vi "Process.vi"(8 "error in":errorcluster, 11 "Measurement.Free":refnum<class "Measurement.Free.lvclass">) -> (0 "error out":errorcluster, 3 "Measurement.Free out":refnum<class "Measurement.Free.lvclass">)   [LabVIEW 2017, in "Measurement.Free.lvclass"]
doc: "---------------------------------------------------------------\nJKI State Machine Objects™\nhttp://jki.net/state-machine-objects/\nCopyright (C) 2005-2015, JKI <info@jki.net>\nALL RIGHTS RESERVEDJKI State Machine Objects (SMO) 1.0.0.5\nJKI - JKI\nCopyright (c) 2016, JKI"
uses:
  Measurement.Free.lvclass
  D:/Program Files (x86)/National Instruments/LabVIEW 2017/vi.lib/JKI/JKI SMO/SMO/SMO.lvclass
  D:/upwork/Laser Measurement Tool/Laser/project/Subsystems/Measurement/Measurement.lvclass
  <vilib>/JKI/JKI SMO/SMO/Typedefs/SMOState --Enum.ctl
  <vilib>/JKI/JKI SMO/SMO/Typedefs/Parent Call--Enum.ctl
  Measurement/Typedefs/Measurement.State--Enum.ctl
  Typedefs/Measurement.Free.Device--Enum.ctl
  Typedefs/Measurement.Free.Measured--Data.ctl
  OPA/Typedefs/OPA.Parameter--Enum.ctl
  Measurement/Typedefs/PublicEvents--Measurement.Initialized.ctl
  Measurement/Typedefs/PublicEvents--Measurement.Escaped.ctl
  SMU/SMU.lvclass
  D:/upwork/Laser Measurement Tool/Laser/project/Subsystems/MeasuringDevice/MeasuringDevice.lvclass
  LIA/LIA.lvclass
  OPM/OPM.lvclass
  Measurement/Measurement.lvclass
  <vilib>/JKI/JKI SMO/SMO/SMO.lvclass
  MeasuringDevice/MeasuringDevice.lvclass
  OPA/OPA.lvclass
panel:
  out "LIA GUID":string
  out "SMU GUID":string
  out "LIA Name":string
  out "SMU Name":string
  out "LIA State":T1
  out "SMU State":T1
  # "Measurement.Free\nProcess.vi"
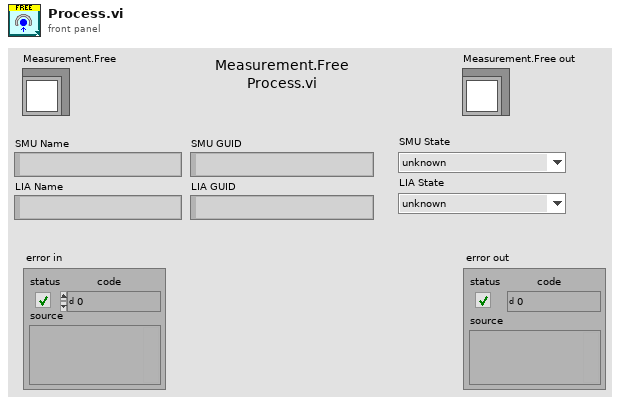
[diagram p1: front panel]
types:
  T1 = typedef "SMO.lvclass/SMOState --Enum.ctl" = enum16{"unknown", "Created", "Started", "Stopped"}
  T2 = typedef "SMO.lvclass/Parent Call--Enum.ctl" = enum16{"Allows parent to run", "Does not request parent to run"}
  T3 = typedef "Measurement.lvclass/Measurement.State--Enum.ctl" = enum16{"Uninitialized", "Initialized", "Started", "Paused", "Stopped"}
  T4 = typedef "Measurement.Free.lvclass/Measurement.Free.Device--Enum.ctl" = enum16{"SMU", "LIA", "OPM", "OPA"}
  T5 = enum32{"invalid app kind", "Development System", "Run Time System", "Student Edition", "Embedded LabVIEW", "Evaluation", "Custom"}
  T6 = enum32{"Invalid", "Standard", "Closed", "Hidden", "Minimized", "Maximized"}
  T7 = typedef "Measurement.lvclass/PublicEvents--Measurement.Initialized.ctl" = bool
  T8 = typedef "Measurement.lvclass/PublicEvents--Measurement.Escaped.ctl" = bool
  T9 = typedef "Measurement.Free.lvclass/Dependencies--Cluster.ctl" = cluster{"SMU":refnum<class "SMU.lvclass">, "LIA":refnum<class "LIA.lvclass">, "OPM":refnum<class "OPM.lvclass">, "OPA":refnum<class "OPA.lvclass">}
  T10 = typedef "Measurement.Free.lvclass/Configuration--Cluster.ctl" = cluster{"Measurement.Type":T11, "Hardware":T12}
  T11 = typedef "Measurement.lvclass/Measurement.Type--Enum.ctl" = enum16{"Free", "I/V Curve", "Wavelength sweeping", "Photocurrent mapping"}
  T12 = typedef "Measurement.Free.lvclass/Configuration.Hardware--Cluster.ctl" = cluster{"SMU":T13, "LIA":T15, "OPM":T17, "OPA":T19}
  T13 = typedef "Measurement.lvclass/Configuration.SMU--Cluster.ctl" = cluster{"Enable":bool, "SMU Model":string, "Configuration":T14}
  T14 = typedef "SMU.lvclass/Configuration--Cluster.ctl" = cluster{"VISA Resource":string, "Channel":string}
  T15 = typedef "Measurement.lvclass/Configuration.LIA--Cluster.ctl" = cluster{"Enable":bool, "LIA Model":string, "Configuration":T16}
  T16 = typedef "LIA.lvclass/Configuration--Cluster.ctl" = cluster{"VISA Resource":string}
  T17 = typedef "Measurement.lvclass/Configuration.OPM--Cluster.ctl" = cluster{"Enable":bool, "OPM Model":string, "Configuration":T18}
  T18 = typedef "OPM.lvclass/Configuration--Cluster.ctl" = cluster{"VISA Resource":string}
  T19 = typedef "Measurement.lvclass/Configuration.OPA--Cluster.ctl" = cluster{"Enable":bool, "OPA Model":string, "Configuration":T20}
  T20 = typedef "OPA.lvclass/Configuration--Cluster.ctl" = cluster{"Serial Number":string}
  T21 = cluster{"Core":cluster{"Current VI Reference":refnum<vi>, "Close Panel on Exit?":bool, "error":errorcluster}, "Self Reference":refnum<class "Measurement.Free.lvclass">, "Dependencies":T9, "Configuration":T10, "Initialized":bool, "State":T3, "SMU Completed":bool, "LIA Completed":bool, "OPM Completed":bool}
  T22 = typedef "Measurement.Free.lvclass/PrivateEvents--Measurement.Free.SMU.SetVoltage.ctl" = dbl
  T23 = typedef "Measurement.Free.lvclass/PrivateEvents--Measurement.Free.OPA.SetWavelength.ctl" = dbl
  T24 = typedef "Measurement.Free.lvclass/PrivateEvents--Measurement.Free.OPA.SetShutterState.ctl" = bool
  T25 = typedef "Measurement.Free.lvclass/Measurement.Free.Measured--Data.ctl" = cluster{"Device":T4, "Parameter":variant, "Data":variant}
  T26 = typedef "OPA.lvclass/OPA.Parameter--Enum.ctl" = enum16{"Wavelength", "Shutter State"}
  T27 = cluster{"Current VI Reference":refnum<vi>, "Close Panel on Exit?":bool, "error":errorcluster}
  T28 = typedef "SMO.lvclass/Protected Events.ctl" = cluster{"StopProcesses":refnum<user-event>, "AbortProcesses":refnum<user-event>, "Config Changed":refnum<user-event>, "Dependency":refnum<user-event>}
  T29 = typedef "Measurement.Free.lvclass/PrivateEvents--Cluster.ctl" = cluster{"SMU.SetVoltage":refnum<user-event>, "OPA.SetWavelength":refnum<user-event>, "OPA.SetShutterState":refnum<user-event>}
  T30 = typedef "SMO.lvclass/Public Events.ctl" = cluster{"Error":refnum<user-event>, "State":refnum<user-event>, "Reserve State":refnum<user-event>}
  T31 = cluster{"Event Registration Refnum":refnum<event-registration>, "Measurement Protected Events":refnum<event-registration>, "SMU Public Events":refnum<event-registration>, "LIA Public Events":refnum<event-registration>, "OPM Public Events":refnum<event-registration>, "OPA Public Events":refnum<event-registration>}
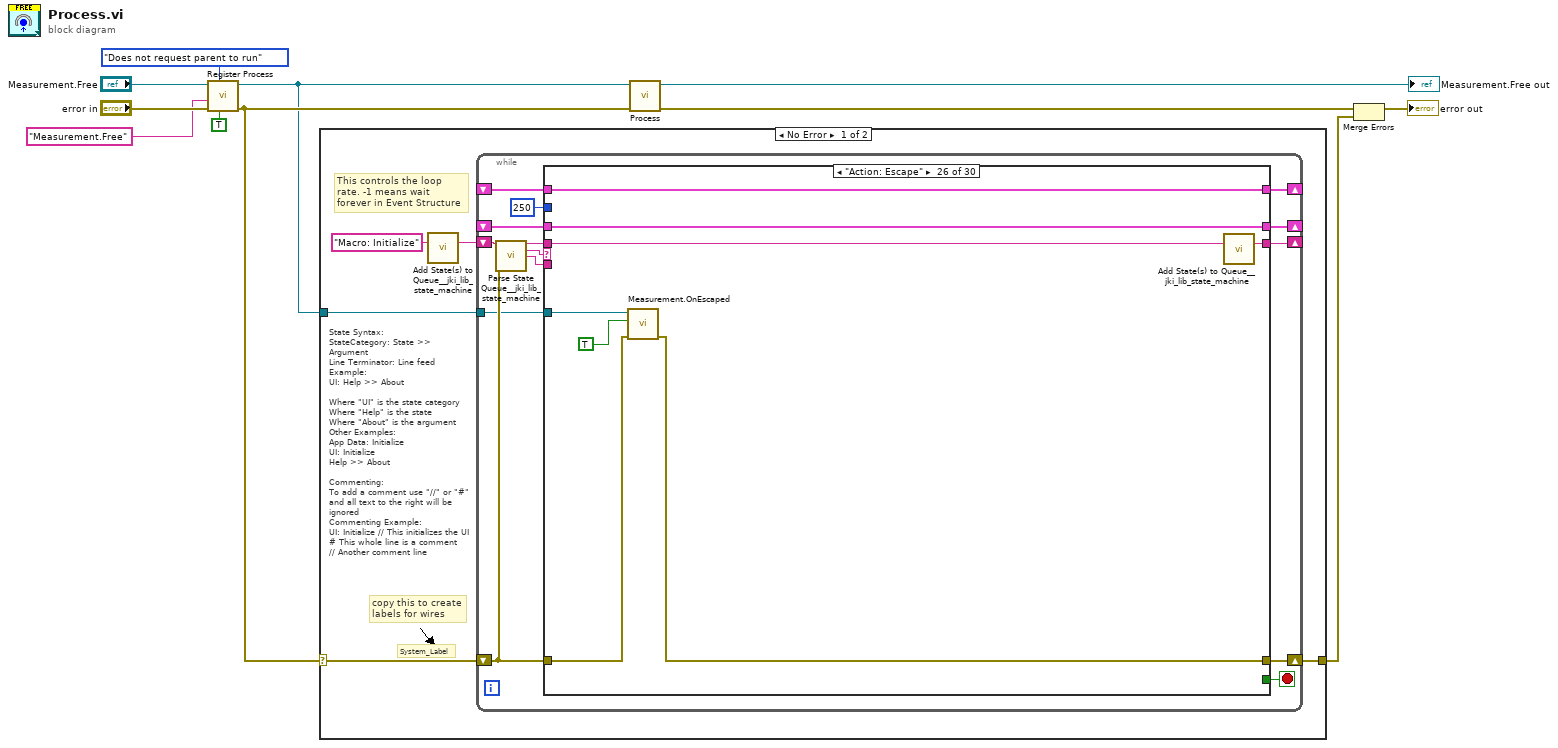
[diagram p0: block diagram]
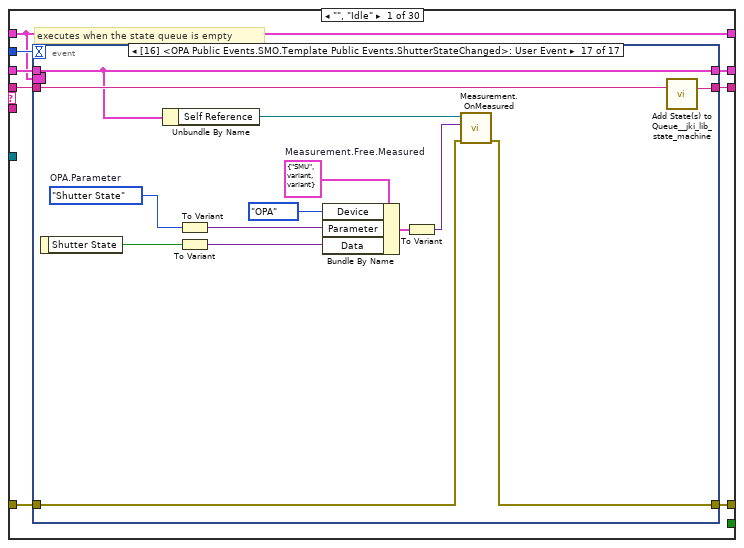
[diagram p2: hidden frame]
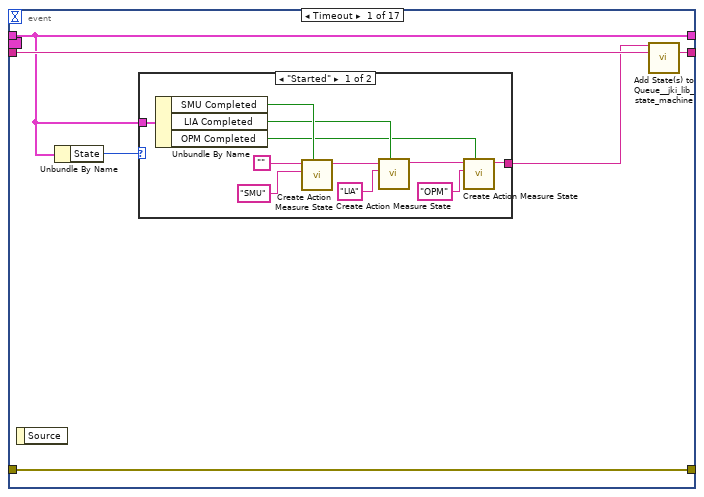
[diagram p3: hidden frame]
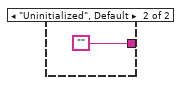
[diagram p4: hidden frame]
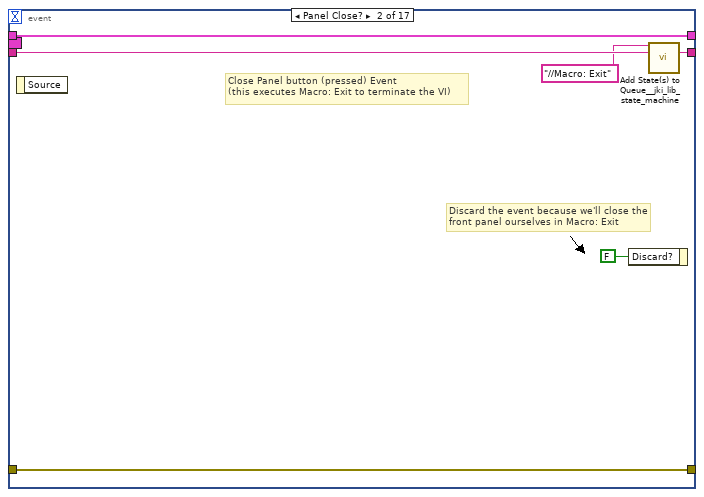
[diagram p5: hidden frame]
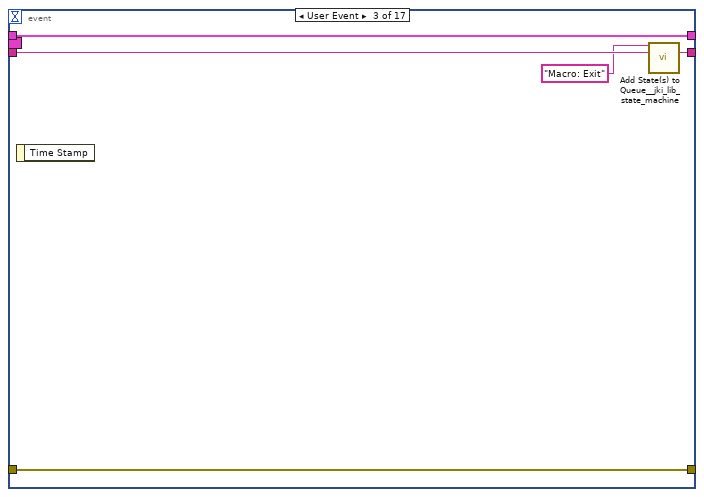
[diagram p6: hidden frame]
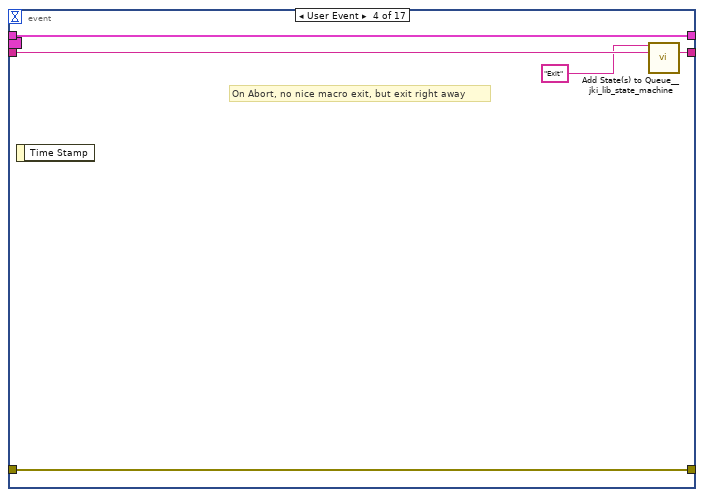
[diagram p7: hidden frame]
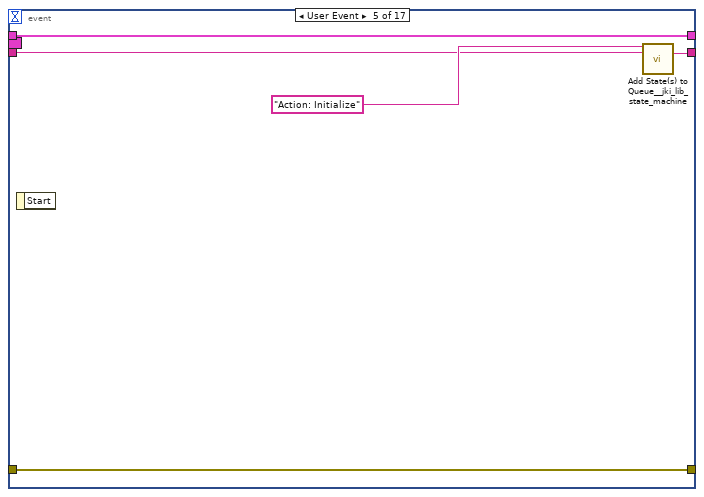
[diagram p8: hidden frame]
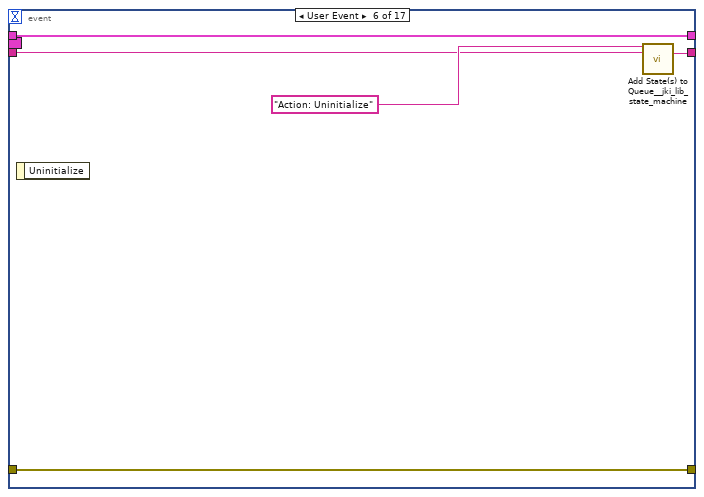
[diagram p9: hidden frame]
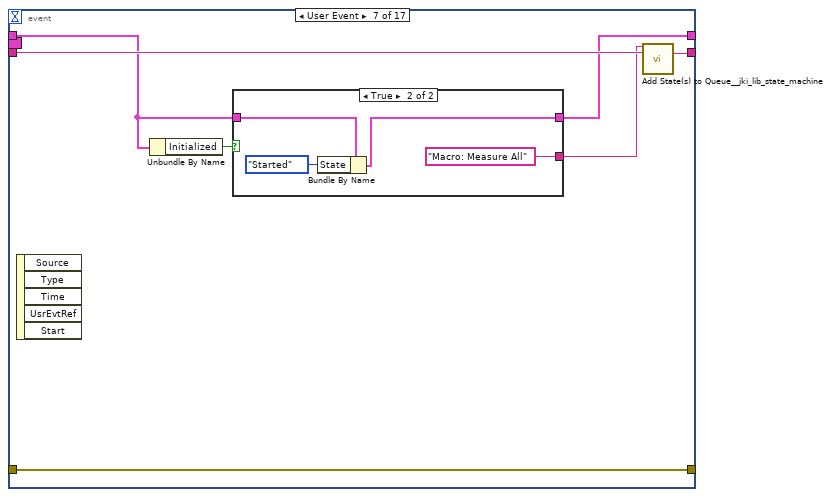
[diagram p10: hidden frame]
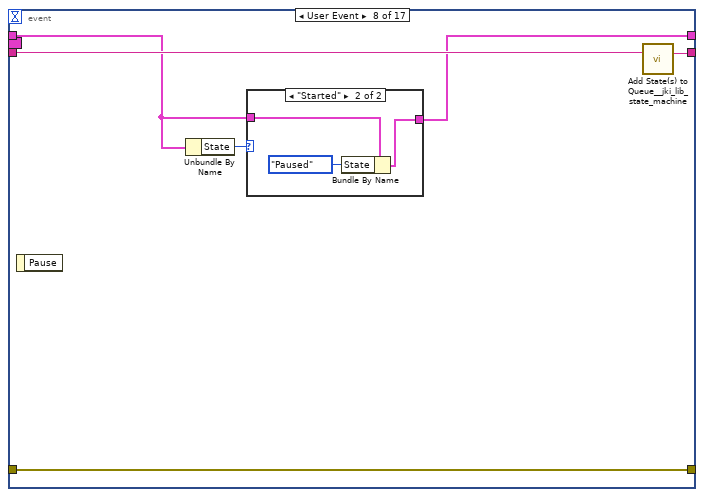
[diagram p12: hidden frame]
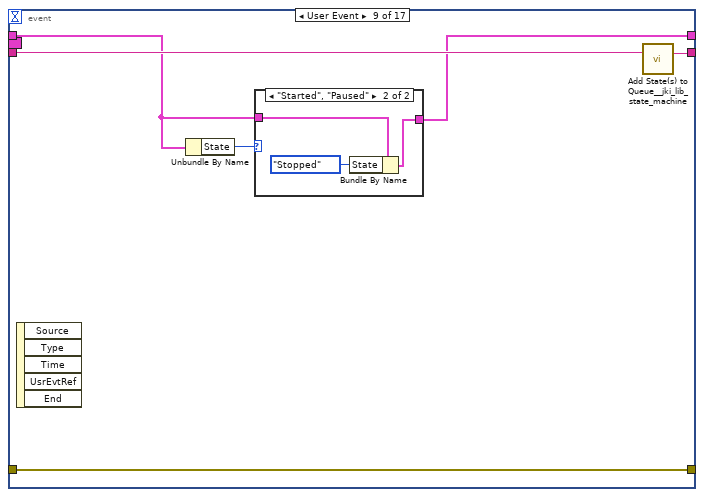
[diagram p14: hidden frame]
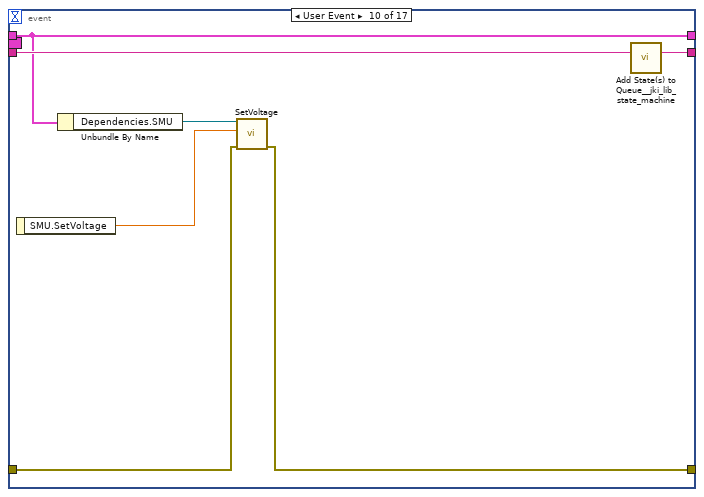
[diagram p16: hidden frame]
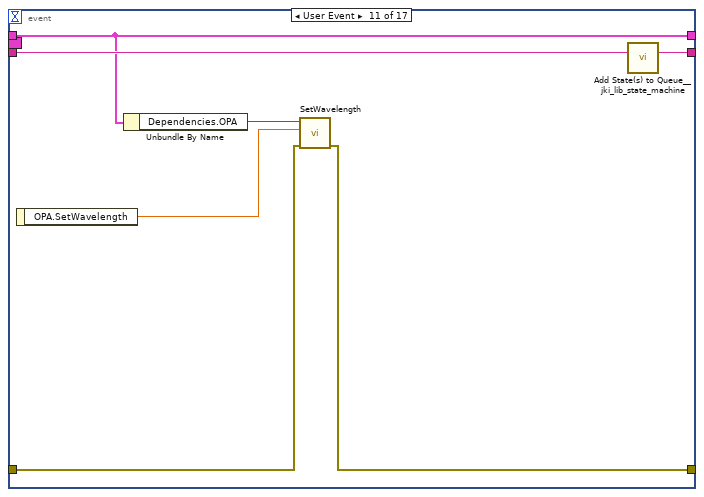
[diagram p17: hidden frame]
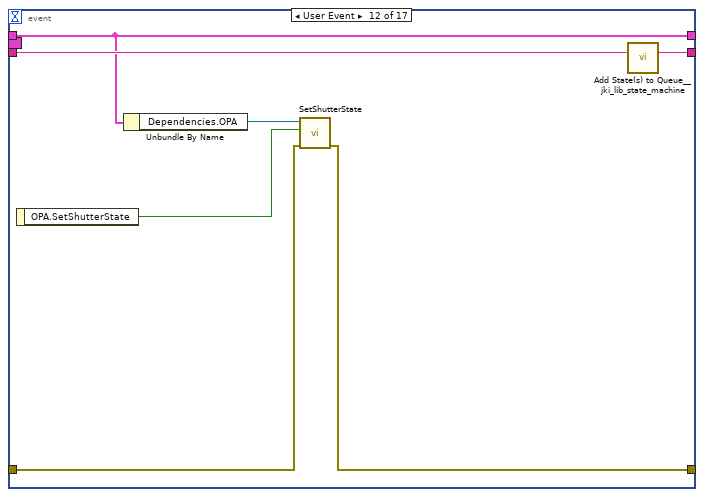
[diagram p18: hidden frame]
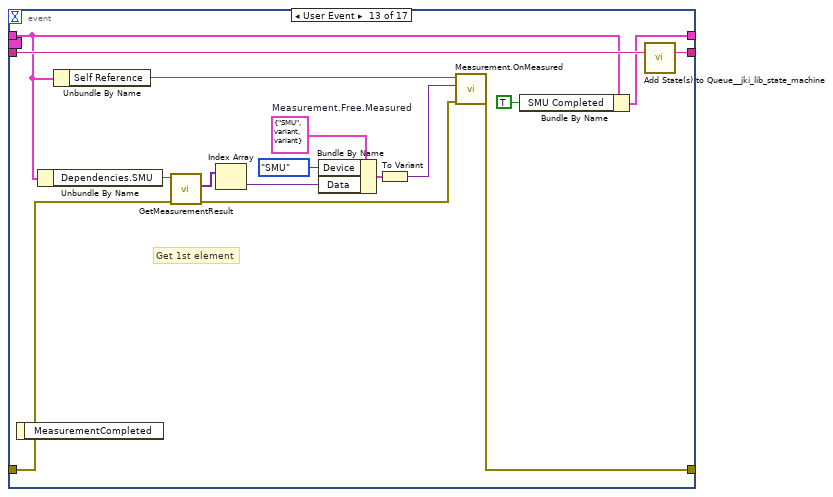
[diagram p19: hidden frame]
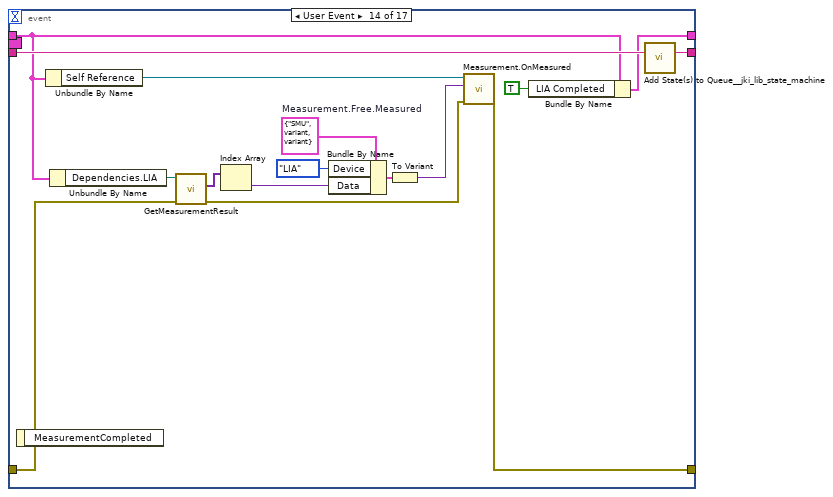
[diagram p20: hidden frame]
diagram:
  n1 = call <vilib>:"Register Process.vi"("Forces Self to Run (F)"=TRUE, "Parent Call"=Parent_Call--Enum."Does not request parent to run", "error in (no error)"="error in", "Process Name (optional)"="Measurement.Free", "SMO"="Measurement.Free") -> ("error out"=w8:errorcluster, "SMO out"=w7:refnum<class "Measurement.Free.lvclass">)  [unwired: 5 in]
  n2 = case shown="No Error" w8 {
    selector: w8 -> [w13 w570]
    tunnel: w7 -> [w14 _]
    tunnel: [w12 w570] -> w4
    frame No Error {
      # "State Syntax:\nStateCategory: State >> Argument\nLine Terminator: Line feed\nExample:\nUI: Help >> About\n\nWhere \"UI\" is the state category\nWhere \"Help\" is the state\nWhere \"About\" is the argument\nOther Examples:\nApp Data: Initialize\nUI: Initialize\nHelp >> About\n\nCommenting:\nTo add a comment use \"//\" or \"#\" and all text to the right will be ignored\nCommenting Example:\nUI: Initialize // This initializes the UI\n# This whole line is a comment\n// Another comment line"
      # "copy this to create labels for wires"
      # "This controls the loop rate. -1 means wait forever in Event Structure"
      # "System_Label"
      n3 = call <vilib>:"Add State(s) to Queue__jki_lib_state_machine.vi"("State(s) in (\"\")"="Macro: Initialize") -> ("States Out"=w16:string)  [unwired: 14 in]
      n4 = while {
        shift-right: [w23] -> _
        shift-left: _ -> [w22]
        shift-right: [w26] -> w12
        shift-left: w13 -> [w20]
        shift-right: [w25] -> _
        shift-left: w16 -> [w27]
        tunnel: w14 -> [w19]
        shift-right: [w18] -> _
        shift-left: _ -> [w17]
        stop <- w24 stop-if-true
        n5 = call <vilib>:"Parse State Queue__jki_lib_state_machine.vi"("State Queue"=w27, "Error In (no error)"=w20) -> ("Remaining States"=w29:string, "Current State"=w30:string, "Arguments"=w28:string)  [unwired: 11 in]
        n6 = case shown="\"Action: Escape\"" w30 {
          selector: w30 -> [_ _ w218 _ _ _ _ _ _ _ _ _ _ _ _ _ _ _ _ _ _ _ _ _ _ _ _ _ _ _]
          tunnel: w29 -> [w38 w216 w222 w241 w256 w262 w267 w287 w294 w299 w304 w311 w327 w359 w368 w383 w397 w402 w413 w418 w451 w457 w462 w475 w493 w508 w518 w528 w538 w566]
          tunnel: w28 -> [_ _ _ _ _ _ _ _ _ _ _ w305 w321 _ _ _ _ _ _ _ _ _ _ _ _ _ _ _ _ _]
          tunnel: w22 -> [w36 w213 w220 w232 w247 w258 w264 _ w289 w296 w302 w309 w323 w356 w364 w372 w388 w399 w410 w415 w422 w455 w460 w469 w484 w505 w510 w521 w531 w549]
          tunnel: [w35 w214 w224 w238 w249 w257 w265 w270 w290 w297 w301 w306 w324 w357 w366 w381 w395 w400 w404 w416 w447 w453 w458 w465 w485 w502 w513 w523 w533 w541] -> w26
          tunnel: w20 -> [w34 w214 w223 w238 w244 _ w265 w284 w291 w297 w301 w307 w325 w357 w366 w381 w395 w400 w405 w416 w448 w453 w458 w471 w489 w503 w512 w522 w532 w548]
          tunnel: [w37 w215 w221 w240 w255 w261 w266 w286 w293 w298 w303 w310 w326 w358 w367 w382 w396 w401 w412 w417 w450 w456 w461 w474 w492 w507 w517 w527 w537 w565] -> w25
          tunnel: [_ _ _ _ _ TRUE _ _ _ _ _ _ _ _ _ _ _ _ _ _ _ _ _ _ _ _ _ _ _ _] -> w24
          tunnel: [w33 w213 w220 w239 w246 w258 w264 w285 w289 w296 w302 w309 w323 w356 w364 w372 w388 w399 w410 w415 w422 w455 w460 w468 w488 w505 w509 w520 w530 w549] -> w23
          tunnel: 250 ("Timeout") -> [w32 _ _ _ _ _ _ _ _ _ _ _ _ _ _ _ _ _ _ _ _ _ _ _ _ _ _ _ _ _]
          tunnel: w19 -> [_ _ _ _ _ _ _ w282 _ _ _ _ _ _ _ _ _ _ _ _ _ _ _ w472 w490 w504 _ _ _ _]
          tunnel: [w31 w212 w217 w229 w254 w259 w263 w281 w288 w295 w300 w308 w320 w355 w365 w380 w389 w398 w411 w414 w438 w454 w459 w473 w491 w506 w516 w526 w536 w564] -> w18
          tunnel: w17 -> [w31 w212 w217 w229 w254 w259 w263 w281 w288 w295 w300 w308 w320 w355 w365 w380 w389 w398 w411 w414 _ w454 w459 w473 w491 w506 w516 w526 w536 w564]
          frame "", "Idle" {
            # "executes when the state queue is empty"
            n7 = event shown="[16] <OPA Public Events.SMO.Template Public Events.ShutterStateChanged>: User Event" {
              selector: w31 -> [_ _ _ _ _ _ _ _ _ _ _ _ _ _ _ _ _]
              dyn-events: _ -> [_ _ _ _ _ _ _ _ _ _ _ _ _ _ _ _ _]
              timeout: w32 -> [_ _ _ _ _ _ _ _ _ _ _ _ _ _ _ _ _]
              tunnel: w38 -> [w44 w62 w67 w72 w75 w80 w88 w99 w109 w120 w127 w134 w150 w166 w182 w196 w210]
              tunnel: [w43 w61 w66 w71 w76 w81 w89 w100 w110 w121 w128 w135 w151 w167 w183 w197 w211] -> w37
              tunnel: w36 -> [w40 w59 w64 w69 w74 w79 w86 w96 w106 w119 w126 w133 w144 w159 w176 w194 w208]
              tunnel: [w42 w60 w65 w70 w73 w78 w87 w98 w108 w115 w122 w130 w145 w161 w177 w192 w206] -> w35
              tunnel: w34 -> [w42 w60 w65 w70 w73 w78 w87 w98 w108 w116 w123 w131 w148 w164 w180 w193 w207]
              tunnel: [w40 w59 w64 w69 w74 w79 w85 w95 w105 w119 w126 w133 w142 w158 w175 w194 w208] -> w33
              event Timeout {
                n8 = event-data() -> ()  [unwired: 1 in, 1 out]
                n9 = Unbundle By Name(w40) -> ("State"=w41:T3)
                n10 = case shown="\"Started\"" w41 {
                  tunnel: w40 -> [w55 _]
                  tunnel: [w52 ""] -> w39
                  frame "Started" {
                    n11 = Unbundle By Name(w55) -> ("SMU Completed"=w51:bool, "LIA Completed"=w50:bool, "OPM Completed"=w49:bool)
                    n12 = call "Create Action Measure State.vi"("Enable"=w51, "Device"="SMU", "States in"="") -> ("States out"=w54:string)  [unwired: 8 in]
                    n13 = call "Create Action Measure State.vi"("Enable"=w50, "Device"="LIA", "States in"=w54) -> ("States out"=w53:string)  [unwired: 8 in]
                    n14 = call "Create Action Measure State.vi"("Enable"=w49, "Device"="OPM", "States in"=w53) -> ("States out"=w52:string)  [unwired: 8 in]
                  }
                  frame "Uninitialized", Default {
                  }
                }
                n15 = call <vilib>:"Add State(s) to Queue__jki_lib_state_machine.vi"("State(s) in Front (\"\")"=w39, "State(s) in (\"\")"=w44) -> ("States Out"=w43:string)  [unwired: 13 in]
              }
              event Panel Close? {
                # "Discard the event because we'll close the front panel ourselves in Macro: Exit"
                # "Close Panel button (pressed) Event\n(this executes Macro: Exit to terminate the VI)"
                n16 = event-data() -> ()  [unwired: 1 in, 1 out]
                n17 = event-data("Discard?"=FALSE) -> ()  [unwired: 1 in, 1 out]
                n18 = call <vilib>:"Add State(s) to Queue__jki_lib_state_machine.vi"("State(s) in Front (\"\")"="//Macro: Exit", "State(s) in (\"\")"=w62) -> ("States Out"=w61:string)  [unwired: 13 in]
              }
              event User Event {
                n19 = event-data() -> ()  [unwired: 1 in, 1 out]
                n20 = call <vilib>:"Add State(s) to Queue__jki_lib_state_machine.vi"("State(s) in Front (\"\")"="Macro: Exit", "State(s) in (\"\")"=w67) -> ("States Out"=w66:string)  [unwired: 13 in]
              }
              event User Event {
                # "On Abort, no nice macro exit, but exit right away"
                n21 = event-data() -> ()  [unwired: 1 in, 1 out]
                n22 = call <vilib>:"Add State(s) to Queue__jki_lib_state_machine.vi"("State(s) in Front (\"\")"="Exit", "State(s) in (\"\")"=w72) -> ("States Out"=w71:string)  [unwired: 13 in]
              }
              event User Event {
                n23 = event-data() -> ()  [unwired: 1 in, 1 out]
                n24 = call <vilib>:"Add State(s) to Queue__jki_lib_state_machine.vi"("State(s) in Front (\"\")"="Action: Initialize", "State(s) in (\"\")"=w75) -> ("States Out"=w76:string)  [unwired: 13 in]
              }
              event User Event {
                n25 = event-data() -> ()  [unwired: 1 in, 1 out]
                n26 = call <vilib>:"Add State(s) to Queue__jki_lib_state_machine.vi"("State(s) in Front (\"\")"="Action: Uninitialize", "State(s) in (\"\")"=w80) -> ("States Out"=w81:string)  [unwired: 13 in]
              }
              event User Event {
                n27 = event-data() -> ()  [unwired: 1 in, 5 out]
                n28 = Unbundle By Name(w86) -> ("Initialized"=w84:bool)
                n29 = case shown="True" w84 {
                  tunnel: w86 -> [w90 w94]
                  tunnel: [w90 w92] -> w85
                  tunnel: [_ "Macro: Measure All"] -> w83
                  frame False {
                  }
                  frame True {
                    n30 = Bundle By Name(cluster=w94, "State"=Measurement.State--Enum."Started") -> (w92:T21)
                  }
                }
                n31 = call <vilib>:"Add State(s) to Queue__jki_lib_state_machine.vi"("State(s) in Front (\"\")"=w83, "State(s) in (\"\")"=w88) -> ("States Out"=w89:string)  [unwired: 13 in]
              }
              event User Event {
                n32 = event-data() -> ()  [unwired: 1 in, 1 out]
                n33 = Unbundle By Name(w96) -> ("State"=w97:T3)
                n34 = case shown="\"Started\"" w97 {
                  tunnel: w96 -> [w101 w104]
                  tunnel: [w101 w102] -> w95
                  frame "Uninitialized", Default {
                  }
                  frame "Started" {
                    n35 = Bundle By Name(cluster=w104, "State"=Measurement.State--Enum."Paused") -> (w102:T21)
                  }
                }
                n36 = call <vilib>:"Add State(s) to Queue__jki_lib_state_machine.vi"("State(s) in (\"\")"=w99) -> ("States Out"=w100:string)  [unwired: 14 in]
              }
              event User Event {
                n37 = event-data() -> ()  [unwired: 1 in, 5 out]
                n38 = Unbundle By Name(w106) -> ("State"=w107:T3)
                n39 = case shown="\"Started\", \"Paused\"" w107 {
                  tunnel: w106 -> [w111 w114]
                  tunnel: [w111 w112] -> w105
                  frame "Uninitialized", Default {
                  }
                  frame "Started", "Paused" {
                    n40 = Bundle By Name(cluster=w114, "State"=Measurement.State--Enum."Stopped") -> (w112:T21)
                  }
                }
                n41 = call <vilib>:"Add State(s) to Queue__jki_lib_state_machine.vi"("State(s) in (\"\")"=w109) -> ("States Out"=w110:string)  [unwired: 14 in]
              }
              event User Event {
                n42 = event-data() -> ("SMU.SetVoltage"=w117:T22)  [unwired: 1 in]
                n43 = Unbundle By Name(w119) -> ("Dependencies.SMU"=w118:refnum<class "SMU.lvclass">)
                n44 = call "SetVoltage.vi"("error in (no error)"=w116, "Voltage, V"=w117, "SMU in"=w118) -> ("error out"=w115:errorcluster)  [unwired: 7 in, 1 out]
                n45 = call <vilib>:"Add State(s) to Queue__jki_lib_state_machine.vi"("State(s) in (\"\")"=w120) -> ("States Out"=w121:string)  [unwired: 14 in]
              }
              event User Event {
                n46 = event-data() -> ("OPA.SetWavelength"=w124:T23)  [unwired: 1 in]
                n47 = Unbundle By Name(w126) -> ("Dependencies.OPA"=w125:refnum<class "OPA.lvclass">)
                n48 = call "SetWavelength.vi"("error in (no error)"=w123, "Wavelength, nm"=w124, "OPA in"=w125) -> ("error out"=w122:errorcluster)  [unwired: 7 in, 1 out]
                n49 = call <vilib>:"Add State(s) to Queue__jki_lib_state_machine.vi"("State(s) in (\"\")"=w127) -> ("States Out"=w128:string)  [unwired: 14 in]
              }
              event User Event {
                n50 = event-data() -> ("OPA.SetShutterState"=w129:T24)  [unwired: 1 in]
                n51 = Unbundle By Name(w133) -> ("Dependencies.OPA"=w132:refnum<class "OPA.lvclass">)
                n52 = call "SetShutterState.vi"("error in (no error)"=w131, "Shutter State"=w129, "OPA"=w132) -> ("error out"=w130:errorcluster)  [unwired: 7 in, 1 out]
                n53 = call <vilib>:"Add State(s) to Queue__jki_lib_state_machine.vi"("State(s) in (\"\")"=w134) -> ("States Out"=w135:string)  [unwired: 14 in]
              }
              event User Event {
                w138 = T25 {"Device"=enum."SMU", "Parameter"=variant, "Data"=variant}  # Measurement.Free.Measured
                # "Get 1st element"
                n54 = event-data() -> ()  [unwired: 1 in, 1 out]
                n55 = Unbundle By Name(w144) -> ("Dependencies.SMU"=w149:refnum<class "SMU.lvclass">)
                n56 = Unbundle By Name(w144) -> ("Self Reference"=w147:refnum<class "Measurement.Free.lvclass">)
                n57 = call "GetMeasurementResult.vi"("error in (no error)"=w148, "MeasuringDevice in"=w149) -> ("error out"=w146:errorcluster, "Result"=w141:variant[])  [unwired: 7 in, 1 out]
                n58 = Index Array(array=w141) -> (element=w139:variant)  [unwired: 1 in]
                n59 = Bundle By Name(cluster=w138, "Device"=Measurement.Free.Device--Enum."SMU", "Data"=w139) -> (w137:T25)
                n60 = To Variant(anything=w137) -> (Variant=w136:variant)
                n61 = call "Measurement.OnMeasured.vi"("error in (no error)"=w146, "Payload"=w136, "Measurement in"=w147) -> ("error out"=w145:errorcluster)  [unwired: 7 in, 1 out]
                n62 = Bundle By Name(cluster=w144, "SMU Completed"=TRUE) -> (w142:T21)
                n63 = call <vilib>:"Add State(s) to Queue__jki_lib_state_machine.vi"("State(s) in (\"\")"=w150) -> ("States Out"=w151:string)  [unwired: 14 in]
              }
              event User Event {
                w155 = T25 {"Device"=enum."SMU", "Parameter"=variant, "Data"=variant}  # Measurement.Free.Measured
                n64 = event-data() -> ()  [unwired: 1 in, 1 out]
                n65 = Unbundle By Name(w159) -> ("Self Reference"=w163:refnum<class "Measurement.Free.lvclass">)
                n66 = Unbundle By Name(w159) -> ("Dependencies.LIA"=w165:refnum<class "LIA.lvclass">)
                n67 = call "GetMeasurementResult.vi"("error in (no error)"=w164, "MeasuringDevice in"=w165) -> ("error out"=w162:errorcluster, "Result"=w157:variant[])  [unwired: 7 in, 1 out]
                n68 = Index Array(array=w157) -> (element=w153:variant)  [unwired: 1 in]
                n69 = Bundle By Name(cluster=w155, "Device"=Measurement.Free.Device--Enum."LIA", "Data"=w153) -> (w154:T25)
                n70 = To Variant(anything=w154) -> (Variant=w152:variant)
                n71 = call "Measurement.OnMeasured.vi"("error in (no error)"=w162, "Payload"=w152, "Measurement in"=w163) -> ("error out"=w161:errorcluster)  [unwired: 7 in, 1 out]
                n72 = Bundle By Name(cluster=w159, "LIA Completed"=TRUE) -> (w158:T21)
                n73 = call <vilib>:"Add State(s) to Queue__jki_lib_state_machine.vi"("State(s) in (\"\")"=w166) -> ("States Out"=w167:string)  [unwired: 14 in]
              }
              event User Event {
                w171 = T25 {"Device"=enum."SMU", "Parameter"=variant, "Data"=variant}  # Measurement.Free.Measured
                n74 = event-data() -> ()  [unwired: 1 in, 1 out]
                n75 = Unbundle By Name(w176) -> ("Dependencies.OPM"=w181:refnum<class "OPM.lvclass">)
                n76 = Unbundle By Name(w176) -> ("Self Reference"=w179:refnum<class "Measurement.Free.lvclass">)
                n77 = call "GetMeasurementResult.vi"("error in (no error)"=w180, "MeasuringDevice in"=w181) -> ("error out"=w178:errorcluster, "Result"=w173:variant[])  [unwired: 7 in, 1 out]
                n78 = Index Array(array=w173) -> (element=w169:variant)  [unwired: 1 in]
                n79 = Bundle By Name(cluster=w171, "Device"=Measurement.Free.Device--Enum."OPM", "Data"=w169) -> (w170:T25)
                n80 = To Variant(anything=w170) -> (Variant=w168:variant)
                n81 = call "Measurement.OnMeasured.vi"("error in (no error)"=w178, "Payload"=w168, "Measurement in"=w179) -> ("error out"=w177:errorcluster)  [unwired: 7 in, 1 out]
                n82 = Bundle By Name(cluster=w176, "OPM Completed"=TRUE) -> (w175:T21)
                n83 = call <vilib>:"Add State(s) to Queue__jki_lib_state_machine.vi"("State(s) in (\"\")"=w182) -> ("States Out"=w183:string)  [unwired: 14 in]
              }
              event User Event {
                w188 = T25 {"Device"=enum."SMU", "Parameter"=variant, "Data"=variant}  # Measurement.Free.Measured
                w191 = OPA.Parameter--Enum."Wavelength"  # OPA.Parameter
                n84 = event-data() -> ("Wavelength, nm"=w190:dbl)  [unwired: 1 in]
                n85 = To Variant(anything=w191) -> (Variant=w186:variant)
                n86 = To Variant(anything=w190) -> (Variant=w185:variant)
                n87 = Unbundle By Name(w194) -> ("Self Reference"=w195:refnum<class "Measurement.Free.lvclass">)
                n88 = Bundle By Name(cluster=w188, "Device"=Measurement.Free.Device--Enum."OPA", "Parameter"=w186, "Data"=w185) -> (w187:T25)
                n89 = To Variant(anything=w187) -> (Variant=w184:variant)
                n90 = call "Measurement.OnMeasured.vi"("error in (no error)"=w193, "Payload"=w184, "Measurement in"=w195) -> ("error out"=w192:errorcluster)  [unwired: 7 in, 1 out]
                n91 = call <vilib>:"Add State(s) to Queue__jki_lib_state_machine.vi"("State(s) in (\"\")"=w196) -> ("States Out"=w197:string)  [unwired: 14 in]
              }
              event User Event {
                w202 = T25 {"Device"=enum."SMU", "Parameter"=variant, "Data"=variant}  # Measurement.Free.Measured
                w205 = OPA.Parameter--Enum."Shutter State"  # OPA.Parameter
                n92 = event-data() -> ("Shutter State"=w204:bool)  [unwired: 1 in]
                n93 = Unbundle By Name(w208) -> ("Self Reference"=w209:refnum<class "Measurement.Free.lvclass">)
                n94 = To Variant(anything=w205) -> (Variant=w200:variant)
                n95 = To Variant(anything=w204) -> (Variant=w199:variant)
                n96 = Bundle By Name(cluster=w202, "Device"=Measurement.Free.Device--Enum."OPA", "Parameter"=w200, "Data"=w199) -> (w201:T25)
                n97 = To Variant(anything=w201) -> (Variant=w198:variant)
                n98 = call "Measurement.OnMeasured.vi"("error in (no error)"=w207, "Payload"=w198, "Measurement in"=w209) -> ("error out"=w206:errorcluster)  [unwired: 7 in, 1 out]
                n99 = call <vilib>:"Add State(s) to Queue__jki_lib_state_machine.vi"("State(s) in (\"\")"=w210) -> ("States Out"=w211:string)  [unwired: 14 in]
              }
            }
          }
          frame "---------- Core ----------" {
            # "Do not put any code in this frame.\n(it is a separator no-op)"
            n100 = call <vilib>:"Add State(s) to Queue__jki_lib_state_machine.vi"("State(s) in (\"\")"=w216) -> ("States Out"=w215:string)  [unwired: 14 in]
          }
          frame Default {
            w227 = 42 items=["No error", "Argument error", "Memory is full", "Out of zone", "End of file", "File already open", "Generic file I/O error", "File not found", "File permission error", "Disk is full", "Duplicate path", "Too many files open", "System feature not enabled", "Resource file not found", "Cannot add resource", "Resource not found", "Image not found", "Image memory error", "Pen does not exist", "Config type invalid", "Config token not found", "Config parse error", "Config memory error", "Bad external code format", "Bad external code offset", "External code not present", "Null window", "Destroy window error", "Null menu", "Print aborted", "Bad print record", "Print driver error", "Windows error during printing", "Memory error during printing", "Print dialog error", "Generic print error", "Invalid device refnum", "Device not found", "Device parameter error", "Device unit error", "Cannot open device", "Device call aborted", "Generic error", "Cancelled by user", "Object ID too low", "Object ID too high", "Object not in heap", "Unknown heap", "Unknown object (invalid DefProc)", "Unknown object (DefProc not in table)", "Message out of range", "Invalid (null) method", "Unknown message", "Manager call not supported", "Bad address", "Network operation in progress", "Network operation timed out", "Connection is busy", "Network attribute not supported", "Network error", "Address in use", "System out of memory", "Connection aborted", "Connection refused", "Not connected", "Already connected", "Connection closed", "Initialization error (interapplication manager)", "Bad occurrence", "Wait on unbound occurrence handler", "Occurrence queue overflow", "Datalog type conflict", "Unused", "Unrecognized type (interapplication manager)", "Memory corrupt", "Failed to make temporary DLL", "Old CIN version", "Drag socket not found", "Failed to load drop-object", "Failed to register OLE object", "Failed to release OLE object", "Format specifier type mismatch", "Unknown format specifier", "Too few format specifiers", "Too many format specifiers", "Scan failed", "Newer CIN version", "Error converting to variant", "Runtime menu error", "Password tampered", "Variant attribute not found", "Incompatible variant data type", "Event data is not available", "Event Store is not present", "Occurrence is not found", "Event Queue is not created", "Event info is not available", "Refnum passed is NULL", "Error retrieving Class GUID", "Error retrieving CoClass GUID", "Error retrieving TypeLib GUID.", "Bad built application magic bytes.", "Specific driver is different from the specific driver associated with the Logical Name.", "There is no session opened to the class driver.", "Max Error", "MAX - Error with config objects", "MAX - Error loading configuration", "MAX - Group not supported"]
            # "Current State"
            # "Do not delete, rename, or modify this frame.\n(this is used to capture unhandled states and typos)"
            # "Handle mistyped state name (developer tool)"
            n101 = Format Into String(format string="Software Exception: Unhandled State \"%s\"." ("message"), error in=w223, w218) -> (resulting string=w226:string, error out=w225:errorcluster)  [unwired: 1 in]
            n102 = call <vilib>:"Error Cluster From Error Code.vi"("show call chain? (False)"=TRUE, "error in (no error)"=w225, "error message (\"\")"=w226, "error code (0)"=w227) -> ("error out"=w224:errorcluster)  [unwired: 5 in]
            n103 = call <vilib>:"Add State(s) to Queue__jki_lib_state_machine.vi"("State(s) in (\"\")"=w222) -> ("States Out"=w221:string)  [unwired: 14 in]
          }
          frame "Initialize Core Data" {
            # "Do not delete, rename, or modify this frame.\n(this is used to determine panel behavior on exit)"
            # "originally closed?"
            # "exe?"
            # "If panel starts closed or is an EXE, then close it when we exit"
            n104 = property class="VI"() -> ("Front Panel.Open"=w237:bool)  [unwired: 2 in, 2 out]
            n105 = property class="App"() -> ("App.Kind"=w236:T5)  [unwired: 2 in, 2 out]
            n106 = control-ref of="Current VI Reference"() -> (w230:refnum<vi>)
            n107 = Not(x=w237) -> (.not. x?=w234:bool)
            n108 = Equal?(x=w236, y=T5."Run Time System" ("Application:Kind")) -> (x = y?=w233:bool)
            n109 = Or(x=w234, y=w233) -> (x .or. y?=w231:bool)
            n110 = Bundle By Name(cluster=w232, "Core.Current VI Reference"=w230, "Core.Close Panel on Exit?"=w231) -> (w239:T21)
            n111 = call <vilib>:"Add State(s) to Queue__jki_lib_state_machine.vi"("State(s) in (\"\")"=w241) -> ("States Out"=w240:string)  [unwired: 14 in]
          }
          frame "Error Handler" {
            w249 = errorcluster {"status"=FALSE, "code"=0, "source"=""}  # No error
            # "Overwrite this method to handle errors and pass to parent if not handled. Parent will fire a public event if the error is not handled up the chain of classes."
            # "Handle any errors here.\nYou can also output any states to clean-up after errors occur"
            n112 = Unbundle By Name(w247) -> ("Self Reference"=w253:refnum<class "Measurement.Free.lvclass">)
            n113 = call <vilib>:"Simple Error Handler.vi"("error in (no error)"=w244) -> ("error out"=w243:errorcluster)  [unwired: 4 in, 4 out]
            n114 = call-dynamic "Handle Error.vi"("Stop on Unhandled Error (T)"=TRUE, "error in"=w243, "Measurement"=w253) -> ("handling error"=w250:errorcluster, "Unhandled error"=w248:errorcluster)  [unwired: 6 in, 1 out]
            n115 = Bundle By Name(cluster=w247, "Core.error"=w248) -> (w246:T21)
            n116 = Select(t="Action: Uninitialize\nAction: Escape", s=w250, f="") -> (s? t:f=w251:string)
            n117 = call <vilib>:"Add State(s) to Queue__jki_lib_state_machine.vi"("State(s) in Front (\"\")"=w251, "State(s) in (\"\")"=w256) -> ("States Out"=w255:string)  [unwired: 13 in]
          }
          frame "Exit" {
            # "Do not put any code in this frame.\n(No errors that occur here will be handled.)"
            n118 = Unbundle By Name(w258) -> ("Core.error"=w257:errorcluster)
            n119 = call <vilib>:"Add State(s) to Queue__jki_lib_state_machine.vi"("State(s) in (\"\")"=w262) -> ("States Out"=w261:string)  [unwired: 14 in]
          }
          frame "---------- Data ----------" {
            # "Do not put any code in this frame.\n(It is a separator no-op. You can make a copy of this frame to create a new Data frame)"
            n120 = call <vilib>:"Add State(s) to Queue__jki_lib_state_machine.vi"("State(s) in (\"\")"=w267) -> ("States Out"=w266:string)  [unwired: 14 in]
          }
          frame "Data: Initialize" {
            w268 = FALSE  # Initialized
            w273 = Measurement.State--Enum."Uninitialized"  # State
            w274 = FALSE  # OPM Completed
            w275 = FALSE  # LIA Completed
            w276 = FALSE  # SMU Completed
            w280 = T27 {"Current VI Reference"=refnum, "Close Panel on Exit?"=FALSE, "error"={"status"=FALSE, "code"=0, "source"=""}}  # Core
            w283 = refnum<class "Measurement.Free.lvclass"> refnum  # Self Reference
            # "Configuration"
            # "Dependencies"
            # "do not delete - used by framework"
            # "Data names and types of shift register data are defined by this bundle."
            # "Initialize the shift-register data, here.\n(data names are defined by what you wire into the bundle function)"
            n121 = Variant To Data(error in=w284, type=w283, Variant=w282) -> (data=w279:refnum<class "Measurement.Free.lvclass">, error out=w277:errorcluster)
            n122 = call "Measurement.Free.GetStaticDependencies.vi"("error in (no error)"=w277, "Measurement.Free"=w279) -> ("error out"=w271:errorcluster, "Dependencies"=w278:T9, "Measurement.Free out"=w272:refnum<class "Measurement.Free.lvclass">)  [unwired: 7 in]
            n123 = call "Measurement.Free.GetConfiguration.vi"("error in (no error)"=w271, "Measurement.Free"=w272) -> ("error out"=w270:errorcluster, "Configuration"=w269:T10)  [unwired: 7 in, 1 out]
            n124 = Bundle("Core"=w280, "Self Reference"=w279, "Dependencies"=w278, "Configuration"=w269, "Initialized"=w268, "State"=w273, "SMU Completed"=w276, "LIA Completed"=w275, "OPM Completed"=w274) -> (w285:T21)  [unwired: 1 in]
            n125 = call <vilib>:"Add State(s) to Queue__jki_lib_state_machine.vi"("State(s) in (\"\")"=w287) -> ("States Out"=w286:string)  [unwired: 14 in]
          }
          frame "Data: Cleanup" {
            # "Cleanup any data and references, here.\n(this is called automatically, by the Macro: Exit)"
            n126 = Unbundle By Name(w289) -> ("Core.Current VI Reference"=w292:refnum<vi>)
            n127 = Close Reference(reference=w292, error in (no error)=w291) -> (error out=w290:errorcluster)
            n128 = call <vilib>:"Add State(s) to Queue__jki_lib_state_machine.vi"("State(s) in (\"\")"=w294) -> ("States Out"=w293:string)  [unwired: 14 in]
          }
          frame "---------- UI ----------" {
            # "Do not put any code in this frame.\n(It is a separator no-op. You can make a copy of this frame to create a new UI frame)"
            n129 = call <vilib>:"Add State(s) to Queue__jki_lib_state_machine.vi"("State(s) in (\"\")"=w299) -> ("States Out"=w298:string)  [unwired: 14 in]
          }
          frame "UI: Initialize" {
            # "Initialize the User Interface, here.\n(this is called automatically, by the Macro: Init)"
            n130 = call <vilib>:"Add State(s) to Queue__jki_lib_state_machine.vi"("State(s) in (\"\")"=w304) -> ("States Out"=w303:string)  [unwired: 14 in]
          }
          frame "UI: Cursor Set" {
            # "Argument"
            # "Initialize the User Interface, here.\n(this is called automatically, by the Macro: Init)"
            n131 = disable-structure shown="Default" {
              disable-tunnel: w307 -> [w312 w315]
              disable-tunnel: [w312 w314] -> w306
              disable-tunnel: w305 -> [_ w313]
              frame condition #0 {
              }
              frame condition #1 (active) {
                n132 = case shown="\"Idle\", Default" w313 {
                  tunnel: w315 -> [w317 w319]
                  tunnel: [w316 w318] -> w314
                  frame "Idle", Default {
                    n133 = call <vilib>:"Unset Busy.vi"("error in (no error)"=w317) -> ("error out"=w316:errorcluster)  [unwired: 10 in]
                  }
                  frame "Busy" {
                    n134 = call <vilib>:"Set Busy.vi"("error in (no error)"=w319) -> ("error out"=w318:errorcluster)  [unwired: 9 in, 1 out]
                  }
                }
              }
            }
            n135 = call <vilib>:"Add State(s) to Queue__jki_lib_state_machine.vi"("State(s) in (\"\")"=w311) -> ("States Out"=w310:string)  [unwired: 14 in]
          }
          frame "UI: Front Panel State" {
            # "Argument"
            # "Set Front Panel Open or Closed\n(Usage: \"UI: Front Panel State >> Open|Close\")"
            n136 = Unbundle By Name(w323) -> ("Core.Current VI Reference"=w322:refnum<vi>)
            n137 = disable-structure shown="Default" {
              disable-tunnel: w325 -> [w331 w354]
              disable-tunnel: [w330 w354] -> w324
              disable-tunnel: w322 -> [w329 _]
              disable-tunnel: w321 -> [w328 _]
              frame condition #0 (active) {
                n138 = case shown="\"Close\"" w328 {
                  tunnel: w331 -> [w335 w348]
                  tunnel: [w337 w349] -> w330
                  tunnel: w329 -> [w336 w346]
                  frame "Open", Default {
                    n139 = property class="VI"(reference=w336, error in=w335) -> (reference out=w333:refnum<vi>, error out=w334:errorcluster, "FP.State"=w332:T6)
                    n140 = case shown="\"Closed\"" w332 {
                      tunnel: [w340 w343] -> w337
                      tunnel: w334 -> [w339 w343]
                      tunnel: w333 -> [w338 _]
                      frame "Closed" {
                        n141 = invoke class="VI" method="FP.Open"(reference=w338, error in=w339, "Activate"=TRUE, "State"=T6."Standard") -> (error out=w340:errorcluster)  [unwired: 1 in, 4 out]
                      }
                      frame Default {
                      }
                    }
                  }
                  frame "Close" {
                    n142 = property class="VI"(reference=w346, error in=w348) -> (reference out=w345:refnum<vi>, error out=w347:errorcluster, "FP.State"=w344:T6)
                    n143 = case shown="Default" w344 {
                      tunnel: [w350 w353] -> w349
                      tunnel: w347 -> [w350 w352]
                      tunnel: w345 -> [_ w351]
                      frame "Invalid", "Closed" {
                      }
                      frame Default {
                        n144 = invoke class="VI" method="FP.Close"(reference=w351, error in=w352) -> (error out=w353:errorcluster)  [unwired: 1 in, 2 out]
                      }
                    }
                  }
                }
              }
              frame condition #1 {
              }
            }
            n145 = call <vilib>:"Add State(s) to Queue__jki_lib_state_machine.vi"("State(s) in (\"\")"=w327) -> ("States Out"=w326:string)  [unwired: 14 in]
          }
          frame "---------- Macro ----------" {
            # "Do not put any code in this frame.\n(It is a separator no-op. You can make a copy of this frame to create a new Macro frame)"
            n146 = call <vilib>:"Add State(s) to Queue__jki_lib_state_machine.vi"("State(s) in (\"\")"=w359) -> ("States Out"=w358:string)  [unwired: 14 in]
          }
          frame "Macro: Initialize" {
            w362 = "UI: Initialize\n//UI: Front Panel State >> Open"  # UI: Initialize //UI: Front Panel State >> Open
            # "Initialization Macro\n(This is called once, when the VI starts)"
            n147 = call <vilib>:"Add State(s) to Queue__jki_lib_state_machine.vi"("State(s) in Front (\"\")"="Data: Initialize\nInitialize Core Data\nEvents: Register\nAction: Get Dependencies State", "State(s) in (\"\")"="Process: Sync", "State(s) at Back (\"\")"=w362) -> ("States Out"=w361:string)  [unwired: 12 in]
            n148 = call <vilib>:"Add State(s) to Queue__jki_lib_state_machine.vi"("State(s) in Front (\"\")"=w361, "State(s) in (\"\")"=w368) -> ("States Out"=w367:string)  [unwired: 13 in]
          }
          frame "Macro: Measure All" {
            (unwired) "Action: Measure SMU\nAction: Measure LIA\nAction: Measure OPM"
            n149 = Unbundle By Name(w372) -> ("Configuration.Hardware.SMU.Enable"=w371:bool, "Configuration.Hardware.LIA.Enable"=w370:bool, "Configuration.Hardware.OPM.Enable"=w369:bool)
            n150 = call "Create Action Measure State.vi"("Enable"=w371, "Device"="SMU", "States in"="") -> ("States out"=w375:string)  [unwired: 8 in]
            n151 = call "Create Action Measure State.vi"("Enable"=w370, "Device"="LIA", "States in"=w375) -> ("States out"=w374:string)  [unwired: 8 in]
            n152 = call "Create Action Measure State.vi"("Enable"=w369, "Device"="OPM", "States in"=w374) -> ("States out"=w373:string)  [unwired: 8 in]
            n153 = call <vilib>:"Add State(s) to Queue__jki_lib_state_machine.vi"("State(s) in Front (\"\")"=w373, "State(s) in (\"\")"=w383) -> ("States Out"=w382:string)  [unwired: 13 in]
          }
          frame "Macro: Exit" {
            # "Exit Macro\n(This is called once, when the VI exits)"
            n154 = Unbundle By Name(w388) -> ("Core.Close Panel on Exit?"=w394:bool)
            n155 = Select(t="UI: Front Panel State >> Close", s=w394, f="") -> (s? t:f=w391:string)
            n156 = call <vilib>:"Add State(s) to Queue__jki_lib_state_machine.vi"("State(s) in Front (\"\")"="Data: Cleanup\nEvents: Unregister", "State(s) in (\"\")"="Process: Sync", "State(s) at Back (\"\")"="Action: Get Dependencies State\nExit") -> ("States Out"=w385:string)  [unwired: 12 in]
            n157 = call <vilib>:"Add State(s) to Queue__jki_lib_state_machine.vi"("State(s) in (\"\")"=w391, "State(s) at Back (\"\")"=w385) -> ("States Out"=w390:string)  [unwired: 13 in]
            n158 = call <vilib>:"Add State(s) to Queue__jki_lib_state_machine.vi"("State(s) in Front (\"\")"=w390, "State(s) in (\"\")"=w397) -> ("States Out"=w396:string)  [unwired: 13 in]
          }
          frame "---------- Process ----------" {
            # "Template Separator\n(You can make a copy of, or modify, this frame)"
            n159 = call <vilib>:"Add State(s) to Queue__jki_lib_state_machine.vi"("State(s) in (\"\")"=w402) -> ("States Out"=w401:string)  [unwired: 14 in]
          }
          frame "Process: Sync" {
            n160 = Unbundle By Name(w410) -> ("Self Reference"=w406:refnum<class "Measurement.Free.lvclass">)
            n161 = call <vilib>:"WaitOnProcessSync.vi"("error in (no error)"=w405, "SMO"=w406) -> ("error out"=w404:errorcluster, "Don't run?"=w409:bool)  [unwired: 7 in, 1 out]
            n162 = Select(t="Data: Cleanup\nEvents: Unregister\nExit", s=w409, f="") -> (s? t:f=w403:string)
            n163 = call <vilib>:"Add State(s) to Queue__jki_lib_state_machine.vi"("State(s) in Front (\"\")"=w403, "State(s) in (\"\")"=w413) -> ("States Out"=w412:string)  [unwired: 13 in]
          }
          frame "---------- Events ----------" {
            # "Template Separator\n(You can make a copy of, or modify, this frame)"
            n164 = call <vilib>:"Add State(s) to Queue__jki_lib_state_machine.vi"("State(s) in (\"\")"=w418) -> ("States Out"=w417:string)  [unwired: 14 in]
          }
          frame "Events: Register" {
            # "Measurement base\nProtected events"
            # "Static Dependencies\nPublic Events"
            # "Base Class Events (Do not remove)"
            n165 = Unbundle By Name(w422) -> ("Self Reference"=w426:refnum<class "Measurement.Free.lvclass">)
            n166 = Unbundle By Name(w422) -> ("Dependencies.SMU"=w428:refnum<class "SMU.lvclass">)
            n167 = Unbundle By Name(w422) -> ("Dependencies.LIA"=w427:refnum<class "LIA.lvclass">)
            n168 = Unbundle By Name(w422) -> ("Dependencies.OPM"=w436:refnum<class "OPM.lvclass">)
            n169 = Unbundle By Name(w422) -> ("Dependencies.OPA"=w421:refnum<class "OPA.lvclass">)
            n170 = call <vilib>:"GetProtectedEvents.vi"("SMO"=w426) -> ("error out"=w445:errorcluster, "SMO Protected Events"=w449:T28)  [unwired: 8 in, 1 out]
            n171 = call "Measurement.Free.GetPrivateEvents.vi"("Measurement.Free"=w426) -> ("error out"=w424:errorcluster, "Private Events"=w425:T29)  [unwired: 8 in, 1 out]
            n172 = call "Measurement.GetProtectedEventsRegistration.vi"("Measurement in"=w426) -> ("error out"=w429:errorcluster, "Measurement Protected Events"=w423:refnum<event-registration>)  [unwired: 8 in, 1 out]
            n173 = call "SMU.GetPublicEventsRegistration.vi"("SMU"=w428) -> ("error out"=w432:errorcluster, "SMU Public Events"=w437:refnum<event-registration>)  [unwired: 8 in, 1 out]
            n174 = call "LIA.GetPublicEventsRegistration.vi"("LIA"=w427) -> ("error out"=w431:errorcluster, "LIA Public Events"=w435:refnum<event-registration>)  [unwired: 8 in, 1 out]
            n175 = call "OPM.GetPublicEventsRegistration.vi"("PM"=w436) -> ("error out"=w430:errorcluster, "OPM Public Events"=w434:refnum<event-registration>)  [unwired: 8 in, 1 out]
            n176 = call "OPA.GetPublicEventsRegistration.vi"("OPA"=w421) -> ("error out"=w420:errorcluster, "OPA Public Events"=w419:refnum<event-registration>)  [unwired: 8 in, 1 out]
            n177 = call <vilib>:"GetPublicEvents.vi"("SMO"=w428) -> ("error out"=w442:errorcluster, "Public Events"=w441:T30)  [unwired: 8 in, 1 out]
            n178 = call <vilib>:"GetPublicEvents.vi"("SMO"=w427) -> ("error out"=w443:errorcluster, "Public Events"=w440:T30)  [unwired: 8 in, 1 out]
            n179 = register-events(w449, w425, w441, w440) -> (reference out=w439:refnum<event-registration>, error out=w444:errorcluster)  [unwired: 2 in]
            n180 = Merge Errors(w444, w445, w429, w424, w443, w442) -> (w446:errorcluster)
            n181 = Merge Errors(w432, w431, w430, w420) -> (w433:errorcluster)
            n182 = Bundle("Event Registration Refnum"=w439, "Measurement Protected Events"=w423, "SMU Public Events"=w437, "LIA Public Events"=w435, "OPM Public Events"=w434, "OPA Public Events"=w419) -> (w438:T31)  [unwired: 1 in]
            n183 = call <vilib>:"Add State(s) to Queue__jki_lib_state_machine.vi"("State(s) in (\"\")"=w451) -> ("States Out"=w450:string)  [unwired: 14 in]
            n184 = Merge Errors(w433, w448, w446) -> (w447:errorcluster)
          }
          frame "Events: Unregister" {
            n185 = Unregister For Events(event registration refnum=w454, error in=w453) -> (error out=w452:errorcluster)
            n186 = call <vilib>:"Clear Errors.vi"("error in (no error)"=w452) -> ()  [unwired: 5 in, 2 out]
            n187 = call <vilib>:"Add State(s) to Queue__jki_lib_state_machine.vi"("State(s) in (\"\")"=w457) -> ("States Out"=w456:string)  [unwired: 14 in]
          }
          frame "---------- Action ----------" {
            n188 = call <vilib>:"Add State(s) to Queue__jki_lib_state_machine.vi"("State(s) in (\"\")"=w462) -> ("States Out"=w461:string)  [unwired: 14 in]
          }
          frame "Action: Initialize" {
            n189 = call-dynamic "Measurement.Init.vi"("error in (no error)"=w471, "Measurement.Free in"=w472) -> ("error out"=w470:errorcluster, "Result"=w463:bool, "Measurement.Free out"=w467:refnum<class "Measurement.Free.lvclass">)  [unwired: 6 in, 1 out]
            n190 = case shown="False" w463 {
              tunnel: w470 -> [w479 w482]
              tunnel: [w478 w482] -> w466
              frame False {
                n191 = call <vilib>:"Error Cluster From Error Code.vi"("error in (no error)"=w479, "error message (\"\")"="Measurement Initialization failure" ("source"), "error code (0)"=-8000 ("code")) -> ("error out"=w478:errorcluster)  [unwired: 6 in]
              }
              frame True {
              }
            }
            n192 = call "Measurement.OnInitialized.vi"("error in (no error)"=w466, "Initialized"=w463, "Measurement in"=w467) -> ("error out"=w465:errorcluster)  [unwired: 7 in, 1 out]
            n193 = case shown="True" w463 {
              tunnel: [Measurement.State--Enum."Uninitialized" ("State") Measurement.State--Enum."Initialized" ("State")] -> w464
              frame False {
              }
              frame True {
              }
            }
            n194 = Bundle By Name(cluster=w469, "State"=w464, "Initialized"=w463) -> (w468:T21)
            n195 = call <vilib>:"Add State(s) to Queue__jki_lib_state_machine.vi"("State(s) in (\"\")"=w475) -> ("States Out"=w474:string)  [unwired: 14 in]
          }
          frame "Action: Uninitialize" {
            n196 = Unbundle By Name(w484) -> ("Initialized"=w483:bool)
            n197 = case shown="True" w483 {
              tunnel: w490 -> [_ w500]
              tunnel: w489 -> [w494 w499]
              tunnel: [w494 w496] -> w485
              frame False {
              }
              frame True {
                n198 = call-dynamic "Measurement.Uninit.vi"("error in (no error)"=w499, "Measurement.Free in"=w500) -> ("error out"=w498:errorcluster, "Measurement.Free out"=w497:refnum<class "Measurement.Free.lvclass">)  [unwired: 8 in]
                n199 = call "Measurement.OnUninitialized.vi"("error in (no error)"=w498, "Uninitialized (True)"=T7 TRUE ("Uninitialized"), "Measurement in"=w497) -> ("error out"=w496:errorcluster)  [unwired: 7 in, 1 out]
              }
            }
            n200 = Bundle By Name(cluster=w484, "State"=Measurement.State--Enum."Uninitialized", "Initialized"=FALSE) -> (w488:T21)
            n201 = call <vilib>:"Add State(s) to Queue__jki_lib_state_machine.vi"("State(s) in (\"\")"=w493) -> ("States Out"=w492:string)  [unwired: 14 in]
          }
          frame "Action: Escape" {
            n202 = call "Measurement.OnEscaped.vi"("error in (no error)"=w503, "Escaped"=T8 TRUE, "Measurement in"=w504) -> ("error out"=w502:errorcluster)  [unwired: 7 in, 1 out]
            n203 = call <vilib>:"Add State(s) to Queue__jki_lib_state_machine.vi"("State(s) in (\"\")"=w508) -> ("States Out"=w507:string)  [unwired: 14 in]
          }
          frame "Action: Measure SMU" {
            n204 = Unbundle By Name(w510) -> ("Dependencies.SMU"=w515:refnum<class "SMU.lvclass">)
            n205 = call "Measure.vi"("error in (no error)"=w512, "MeasuringDevice"=w515) -> ("error out"=w514:errorcluster)  [unwired: 7 in, 2 out]
            n206 = Bundle By Name(cluster=w510, "SMU Completed"=FALSE) -> (w509:T21)
            n207 = Merge Errors(w514) -> (w513:errorcluster)
            n208 = call <vilib>:"Add State(s) to Queue__jki_lib_state_machine.vi"("State(s) in (\"\")"=w518) -> ("States Out"=w517:string)  [unwired: 14 in]
          }
          frame "Action: Measure LIA" {
            n209 = Unbundle By Name(w521) -> ("Dependencies.LIA"=w525:refnum<class "LIA.lvclass">)
            n210 = call "Measure.vi"("error in (no error)"=w522, "MeasuringDevice"=w525) -> ("error out"=w524:errorcluster)  [unwired: 7 in, 2 out]
            n211 = Bundle By Name(cluster=w521, "LIA Completed"=FALSE) -> (w520:T21)
            n212 = Merge Errors(w524) -> (w523:errorcluster)
            n213 = call <vilib>:"Add State(s) to Queue__jki_lib_state_machine.vi"("State(s) in (\"\")"=w528) -> ("States Out"=w527:string)  [unwired: 14 in]
          }
          frame "Action: Measure OPM" {
            n214 = Unbundle By Name(w531) -> ("Dependencies.OPM"=w535:refnum<class "OPM.lvclass">)
            n215 = call "Measure.vi"("error in (no error)"=w532, "MeasuringDevice"=w535) -> ("error out"=w534:errorcluster)  [unwired: 7 in, 2 out]
            n216 = Bundle By Name(cluster=w531, "OPM Completed"=FALSE) -> (w530:T21)
            n217 = Merge Errors(w534) -> (w533:errorcluster)
            n218 = call <vilib>:"Add State(s) to Queue__jki_lib_state_machine.vi"("State(s) in (\"\")"=w538) -> ("States Out"=w537:string)  [unwired: 14 in]
          }
          frame "Action: Get Dependencies State" {
            n219 = Unbundle By Name(w549) -> ("Self Reference"=w563:refnum<class "Measurement.Free.lvclass">)
            n220 = call "Measurement.Free.GetStaticDependencies.vi"("error in (no error)"=w548, "Measurement.Free"=w563) -> ("error out"=w540:errorcluster, "Dependencies"=w562:T9)  [unwired: 7 in, 1 out]
            n221 = Unbundle By Name(w562) -> ("SMU"=w559:refnum<class "SMU.lvclass">, "LIA"=w556:refnum<class "LIA.lvclass">)
            n222 = Unbundle By Name(w540) -> ("code"=w539:i32)
            n223 = case shown="116" w539 {
              tunnel: [w567 w569] -> w541
              tunnel: w540 -> [w567 w568]
              frame Default {
              }
              frame 116 {
                # "Filter error 116 (flattening error when no deps)"
                n224 = call <vilib>:"Clear Errors.vi"("error in (no error)"=w568) -> ("error out"=w569:errorcluster)  [unwired: 5 in, 1 out]
              }
            }
            n225 = call <vilib>:"Get State.vi"("SMO"=w556) -> ("error out"=w544:errorcluster, "SMO State"=→"LIA State":T1, "SMO out"=w557:refnum<class "LIA.lvclass">)  [unwired: 8 in]
            n226 = call <vilib>:"Get State.vi"("SMO"=w559) -> ("error out"=w547:errorcluster, "SMO State"=→"SMU State":T1, "SMO out"=w561:refnum<class "SMU.lvclass">)  [unwired: 8 in]
            n227 = call <vilib>:"Get Name.vi"("error in (no error)"=w544, "SMO"=w557) -> ("error out"=w545:errorcluster, "Name"=→"LIA Name":string, "SMO out"=w558:refnum<class "LIA.lvclass">)  [unwired: 7 in]
            n228 = call <vilib>:"Get Name.vi"("error in (no error)"=w547, "SMO"=w561) -> ("error out"=w546:errorcluster, "Name"=→"SMU Name":string, "SMO out"=w560:refnum<class "SMU.lvclass">)  [unwired: 7 in]
            n229 = call <vilib>:"Get GUID.vi"("error in (no error)"=w545, "SMO"=w558) -> ("error out"=w542:errorcluster, "GUID"=→"LIA GUID":string)  [unwired: 7 in, 1 out]
            n230 = call <vilib>:"Get GUID.vi"("error in (no error)"=w546, "SMO"=w560) -> ("error out"=w543:errorcluster, "GUID"=→"SMU GUID":string)  [unwired: 7 in, 1 out]
            n231 = call <vilib>:"Clear Errors.vi"("error in (no error)"=w543) -> ()  [unwired: 5 in, 2 out]
            n232 = call <vilib>:"Clear Errors.vi"("error in (no error)"=w542) -> ()  [unwired: 5 in, 2 out]
            n233 = call <vilib>:"Add State(s) to Queue__jki_lib_state_machine.vi"("State(s) in (\"\")"=w566) -> ("States Out"=w565:string)  [unwired: 14 in]
          }
        }
      }
    }
    frame Error {
    }
  }
  n234 = call-parent "Process.vi"("error in"=w8, "SMO"=w7) -> ("error out"=w5:errorcluster, "SMO out"=→"Measurement.Free out":refnum<class "Measurement.Free.lvclass">)  [unwired: 8 in]
  n235 = Merge Errors(w5, w4) -> (→"error out":errorcluster)
